vi "FTW-ProjectManager-ConditionalDisableSymbols-Set.vi"(0 "Project Manager":refnum<class "FTW-ProjectManager.lvclass">, 5 "Target (Root or My Computer)":string(combo)="Root", 7 "Conditional Disable Symbol":string, 9 "Value":string, 11 "error in":errorcluster) -> (4 "Project Manager out":refnum<class "FTW-ProjectManager.lvclass">, 6 "Conditional Disable Symbols out":string, 15 "error out":errorcluster)   [LabVIEW 2012, in "FTW-ProjectManager.lvclass"]
doc: "This VI will add to or modify existing Conditional Disable Symbols. It will not remove existing Conditional Disable Symbols."
uses:
  FTW-ProjectManager.lvclass
  FTW-ProjectManager.lvclass/FTW-ProjectManager.ctl
panel:
  # "Inputs"
  # "Outputs"
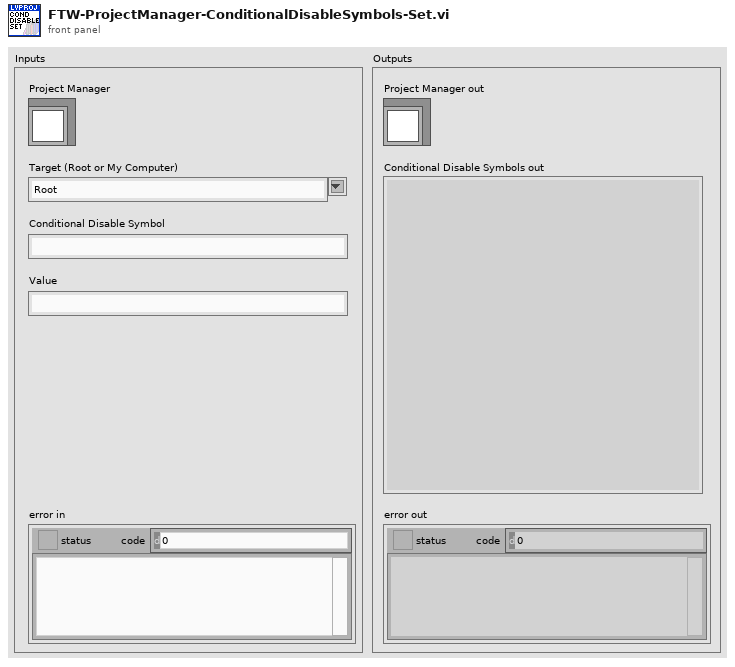
[diagram p1: front panel]
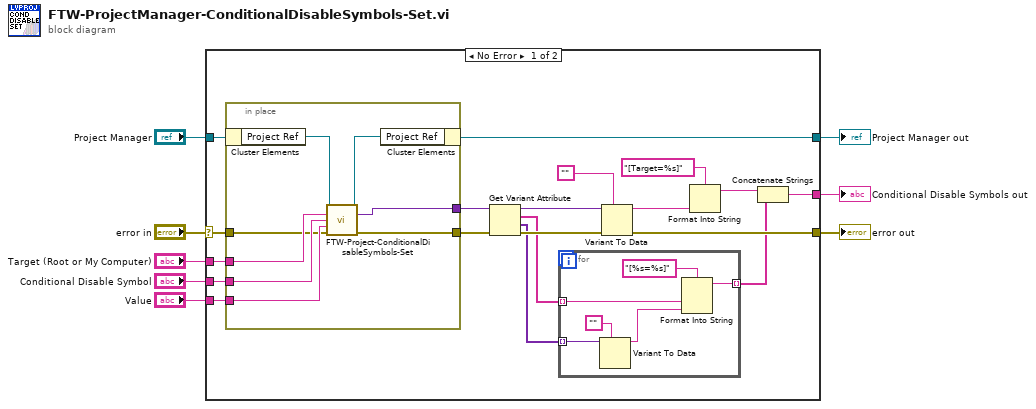
[diagram p0: block diagram]
diagram:
  n1 = case shown="No Error" "error in" {
    selector: "error in" -> [w25 w43]
    tunnel: [w18 w43] -> w8
    tunnel: "Target (Root or My Computer)" -> [w27 _]
    tunnel: [w9 w42] -> w4
    tunnel: "Value" -> [w24 _]
    tunnel: "Conditional Disable Symbol" -> [w26 _]
    tunnel: "Project Manager" -> [w10 w42]
    tunnel: [w11 _] -> w1
    frame No Error {
      n2 = in-place {
        in-place-border: w27 -> [w35]
        in-place-border: w26 -> [w34]
        in-place-border: w25 -> [w30]
        in-place-border: w24 -> [w33]
        in-place-border: [w32] -> w23
        in-place-border: [w31] -> w20
        n3 = in-place-cluster #1(w10) -> ("Project Ref"=w29:refnum<vi>)
        n4 = call "FTW-Project-ConditionalDisableSymbols-Set.vi"("Project Ref (blank for Active Project)"=w29, "Target (Root or My Computer)"=w35, "Conditional Disable Symbol"=w34, "Value"=w33, "error in"=w30) -> ("Project out"=w28:refnum<vi>, "Conditional Disable Symbols out"=w32:variant, "error out"=w31:errorcluster)  [unwired: 8 in]
        n5 = in-place-cluster #1("Project Ref"=w28) -> (w9:refnum<class "FTW-ProjectManager.lvclass">)
      }
      n6 = Get Variant Attribute(Variant=w23, error in=w20) -> (duplicate Variant=w22:variant, names=w17:string[], values=w16:variant[], error out=w19:errorcluster)  [unwired: 2 in]
      n7 = for {
        tunnel: w17 -> [w37] mode=indexing
        tunnel: w16 -> [w41] mode=indexing
        tunnel: [w36] -> w12 mode=indexing
        n8 = Variant To Data(type="", Variant=w41) -> (data=w38:string)  [unwired: 1 in, 1 out]
        n9 = Format Into String(format string="[%s=%s]", w37, w38) -> (resulting string=w36:string)  [unwired: 2 in, 1 out]
      }
      n10 = Variant To Data(error in=w19, type="", Variant=w22) -> (data=w15:string, error out=w18:errorcluster)
      n11 = Format Into String(format string="[Target=%s]", w15) -> (resulting string=w13:string)  [unwired: 2 in, 1 out]
      n12 = Concatenate Strings(w13, w12) -> (w11:string)
    }
    frame Error {
    }
  }
  "error out" <- w8
  "Project Manager out" <- w4
  "Conditional Disable Symbols out" <- w1
